vi "Actor Core.vi"(8 "error in":errorcluster, 11 "Hardware in":refnum<class "scan_2d.lvclass">) -> (0 "error out":errorcluster, 3 "Actor out":refnum<class "Actor.lvclass">)   [LabVIEW 2015, in "scan_2d.lvclass"]
doc: "(<B>Filename</B>: Actor Framework.lvlib:Actor.lvclass:Actor Core.vi)\n\nReceives messages to the actor, reacts to them, and initiates any error handling that may shut the actor down.\n\nDescendant classes may override this VI to append parallel tasks for the actor to complete while it handles messages. Overrides use the Call Parent Method node."
uses:
  scan_2d.lvclass
  <vilib>/ActorFramework/Actor/Actor.lvclass
  UI/panel_class/panel.lvclass/panel.ctl
  scan_2d_settings.ctl
  Scan/scan_record.ctl
  <vilib>/ActorFramework/Actor/Actor.lvclass/Actor.ctl
  <vilib>/ActorFramework/Message Enqueuer/Message Enqueuer.lvclass/Message Enqueuer.ctl
  scan_2d Messages/scan2d_perform_scan Msg/scan2d_perform_scan Msg.lvclass/scan2d_perform_scan Msg.ctl
  <vilib>/ActorFramework/Message Enqueuer/Init from Existing Queue.vi
  <vilib>/ActorFramework/Message Enqueuer/Enqueue.vi
  <vilib>/ActorFramework/Message Priority Queue/Priority Enqueue.vi
  <vilib>/ActorFramework/Message Enqueuer/Message Enqueuer.lvclass
  scan_2d Messages/scan2d_perform_scan Msg/scan2d_perform_scan Msg.lvclass
  UI/panel_class/panel.lvclass
panel:
  in  "notes":string
  in  "copy_bounds":bool
  in  "Y Steps":u32=1
  in  "Y Stop":dbl=0.1
  in  "Y Start":dbl=0.1
  in  "X Steps":u32=1
  in  "X Stop":dbl=0.1
  in  "X Start":dbl=0.1
  in  "scan":bool
  in  "Dwell Time (s)":dbl=0.1 min=0.02
  in  "Save Path":path
  out "Status":string
  in  "Stage Number":enum16{"1", "2"}(ring)=enum."2"
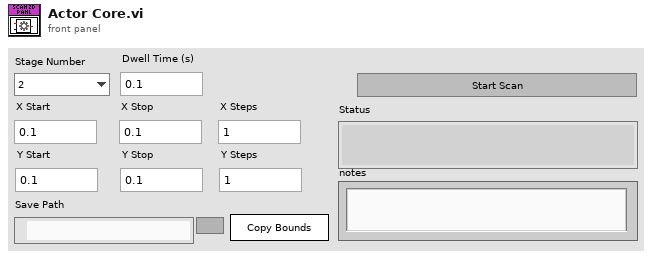
[diagram p1: front panel]
types:
  T1 = cluster{"stop_ui_ref":refnum<event-registration>, "update_status":refnum<event-registration>}
  T2 = typedef "scan_record.ctl" = enum16{"hdf5", "legacy", "None"}
  T3 = typedef "scan_2d_settings.ctl" = cluster{"X Start":dbl, "X Stop":dbl, "X Steps":u32, "Y Start":dbl, "Y Stop":dbl, "Y Steps":u32, "Integration Time":dbl, "Record Type":T2, "Save Path":path, "Stage Number":enum16{"1", "2"}, "notes":string}
  T4 = typedef "ui_plot_references.ctl" = cluster{"plots":refnum<vi>, "chart":refnum<vi>, "graph":refnum<vi>, "map":refnum<vi>, "XY Graph":refnum<vi>}
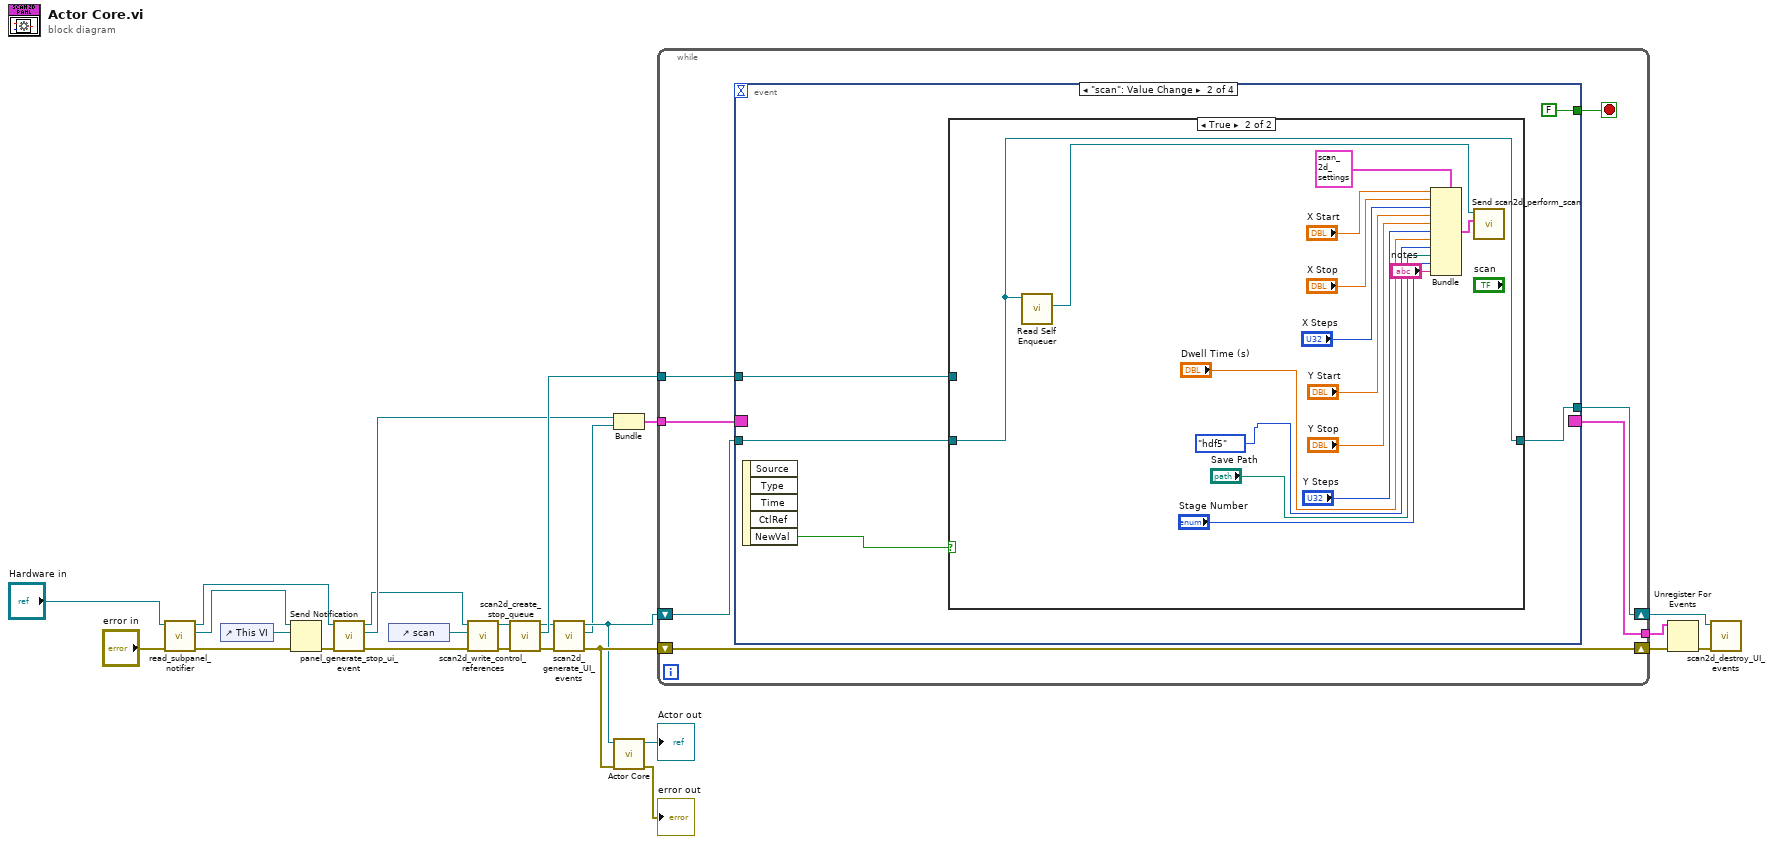
[diagram p0: block diagram]
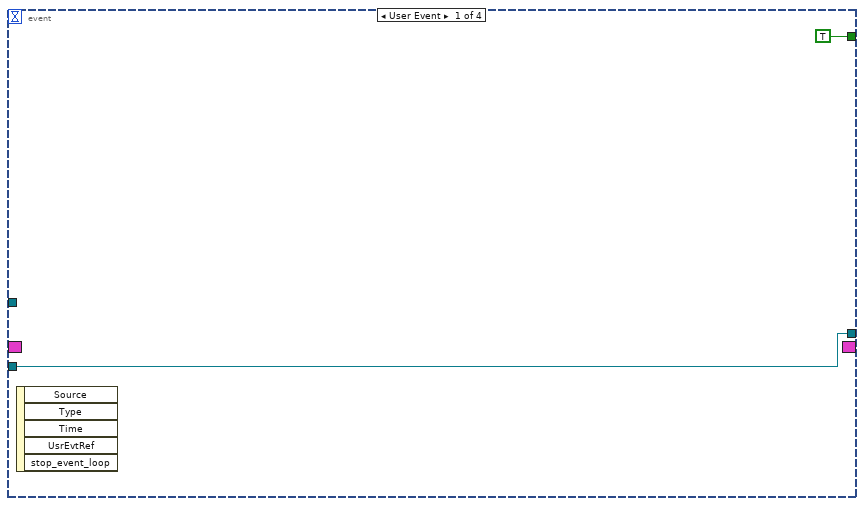
[diagram p2: hidden frame]
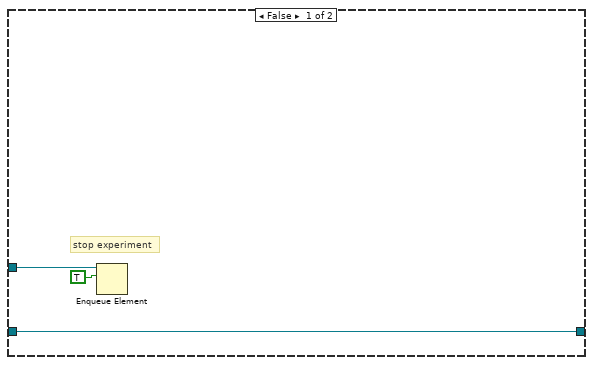
[diagram p3: hidden frame]
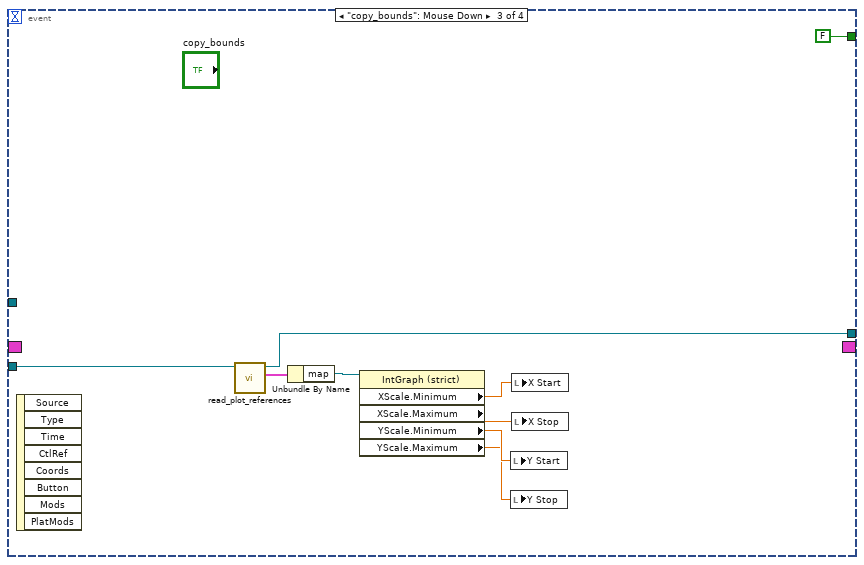
[diagram p4: hidden frame]
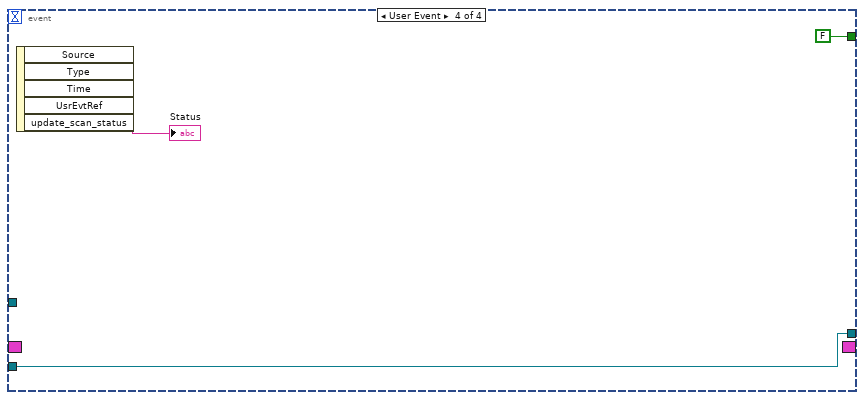
[diagram p5: hidden frame]
diagram:
  n1 = call "read_subpanel_notifier.vi"("error in (no error)"="error in", "panel in"="Hardware in") -> ("error out"=w20:errorcluster, "subpanel_notifier"=w22:refnum<notifier>, "panel out"=w21:refnum<class "scan_2d.lvclass">)  [unwired: 7 in]
  n2 = control-ref of="This VI"() -> (w24:refnum<vi>)
  n3 = Send Notification(notification=w24, notifier=w22, error in (no error)=w20) -> (error out=w19:errorcluster)  [unwired: 1 out]
  n4 = call "panel_generate_stop_ui_event.vi"("error in (no error)"=w19, "panel in"=w21) -> ("error out"=w5:errorcluster, "stop_ui_ref"=w11:refnum<event-registration>, "panel out"=w3:refnum<class "scan_2d.lvclass">)  [unwired: 7 in]
  n5 = control-ref of="scan"() -> (w1:refnum<vi>)
  n6 = call "scan2d_write_control_references.vi"("error in (no error)"=w5, "scan"=w1, "scan_panel in"=w3) -> ("error out"=w4:errorcluster, "scan_panel out"=w2:refnum<class "scan_2d.lvclass">)  [unwired: 7 in]
  n7 = call "scan2d_create_stop_queue.vi"("error in (no error)"=w4, "scan_panel in"=w2) -> ("error out"=w15:errorcluster, "stop_queue"=w16:refnum<queue>, "scan_panel out"=w13:refnum<class "scan_2d.lvclass">)  [unwired: 7 in]
  n8 = call "scan2d_generate_UI_events.vi"("error in (no error)"=w15, "scan_panel in"=w13) -> ("error out"=w14:errorcluster, "update_status"=w10:refnum<event-registration>, "scan_panel out"=w12:refnum<class "scan_2d.lvclass">)  [unwired: 7 in]
  n9 = Bundle("stop_ui_ref"=w11, "update_status"=w10) -> (w9:T1)  [unwired: 1 in]
  n10 = call-parent "Actor Core.vi"("error in"=w14, "Actor in"=w12) -> ("error out"=→"error out":errorcluster, "Actor out"=→"Actor out":refnum<class "Actor.lvclass">)  [unwired: 8 in]
  n11 = while {
    tunnel: w9 -> [w33]
    tunnel: [w31] -> w17
    shift-right: [w30] -> w8
    shift-left: w14 -> [w30]
    tunnel: w16 -> [w29]
    shift-right: [w27] -> w7
    shift-left: w12 -> [w28]
    stop <- w32 stop-if-true
    n12 = event shown="[1] \"scan\": Value Change" {
      selector: w33 -> [_ _ _ _]
      dyn-events: [_ _ _ _] -> w31
      timeout: _ -> [_ _ _ _]
      tunnel: [TRUE FALSE FALSE FALSE] -> w32
      tunnel: w29 -> [_ w38 _ _]
      tunnel: w28 -> [w34 w37 w67 w68]
      tunnel: [w34 w36 w64 w68] -> w27
      event User Event {
        n13 = event-data() -> ()  [unwired: 1 in, 5 out]
      }
      event "scan": Value Change {
        n14 = event-data() -> ("NewVal"=w39:bool)  [unwired: 1 in, 4 out]
        n15 = case shown="True" w39 {
          tunnel: w38 -> [w43 _]
          tunnel: w37 -> [w41 w56]
          tunnel: [w41 w56] -> w36
          frame False {
            # "stop experiment"
            n16 = Enqueue Element(queue=w43, element=TRUE) -> ()  [unwired: 2 in, 3 out]
          }
          frame True {
            n17 = call <vilib>:"Read Self Enqueuer.vi"("Actor"=w56) -> ("Self Enqueuer"=w46:refnum<class "Message Enqueuer.lvclass">)  [unwired: 10 in]
            n18 = Bundle(cluster=T3 {"X Start"=0.0, "X Stop"=0.0, "X Steps"=0, "Y Start"=0.0, "Y Stop"=0.0, "Y Steps"=0, "Integration Time"=0.0, "Record Type"=enum."hdf5", "Save Path"=path "", "Stage Number"=enum."1", "notes"=""} ("output cluster"), "X Start"="X Start", "X Stop"="X Stop", "X Steps"="X Steps", "Y Start"="Y Start", "Y Stop"="Y Stop", "Y Steps"="Y Steps", "Integration Time"="Dwell Time (s)", "Record Type"=scan_record."hdf5", "Save Path"="Save Path", "Stage Number"="Stage Number", "notes"="notes") -> (w47:T3)
            n19 = call "Send scan2d_perform_scan.vi"("scan-2d-settings"=w47, "Message Enqueuer"=w46) -> ()  [unwired: 8 in, 2 out]
          }
        }
      }
      event "copy_bounds": Mouse Down {
        n20 = event-data() -> ()  [unwired: 1 in, 8 out]
        n21 = call "read_plot_references.vi"("panel in"=w67) -> ("plot_references"=w66:T4, "panel out"=w64:refnum<class "scan_2d.lvclass">)  [unwired: 8 in, 1 out]
        n22 = Unbundle By Name(w66) -> ("map"=w65:refnum<vi>)
        n23 = property class="IntGraph (strict)"(reference=w65) -> ("XScale.Minimum"=w62:dbl, "XScale.Maximum"=w61:dbl, "YScale.Minimum"=w60:dbl, "YScale.Maximum"=w59:dbl)  [unwired: 1 in, 2 out]
        n24 = local write "Y Start"(w60) -> ()
        n25 = local write "Y Stop"(w59) -> ()
        n26 = local write "X Start"(w62) -> ()
        n27 = local write "X Stop"(w61) -> ()
      }
      event User Event {
        n28 = event-data() -> ("update_scan_status"=→"Status":string)  [unwired: 1 in, 4 out]
      }
    }
  }
  n29 = Unregister For Events(event registration refnum=w17, error in=w8) -> (error out=w6:errorcluster)
  n30 = call "scan2d_destroy_UI_events.vi"("error in (no error)"=w6, "scan_panel in"=w7) -> ()  [unwired: 8 in, 2 out]
